vi "Calculate Node Width.vi"(11 "ClassInfo":T1[](array[typedef])) -> (3 "upper limit":i16)   [LabVIEW 2016, in "LV Object Event Registration Node.xnode"]
uses:
  LV Object Event Registration Node.xnode
  LOER_ClassInfo.ctl
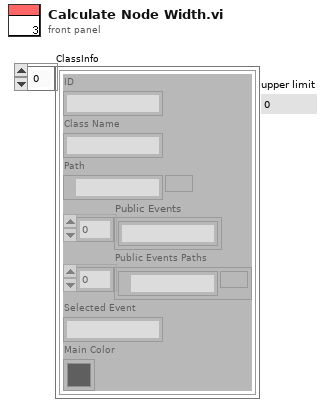
[diagram p1: front panel]
types:
  T1 = typedef "LV Object Event Registration Node.xnode/LOER_ClassInfo.ctl" = cluster{"ID":string, "Class Name":string, "Path":path, "Public Events":string[], "Public Events Paths":path[], "Selected Event":string, "Main Color":u32}
  T2 = cluster{"left":i16, "top":i16, "right":i16, "bottom":i16}
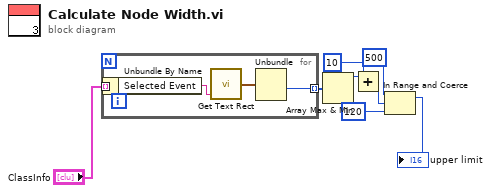
[diagram p0: block diagram]
diagram:
  n1 = for {
    tunnel: "ClassInfo" -> [w11] mode=indexing
    tunnel: [w9] -> w2 mode=indexing
    n2 = Unbundle By Name(w11) -> ("Selected Event"=w10:string)
    n3 = call <vilib>:"Get Text Rect.vi"("text"=w10) -> ("rect"=w12:T2)  [unwired: 8 in]
    n4 = Unbundle(w12) -> ("right"=w9:i16)  [unwired: 3 out]
  }
  n5 = Array Max & Min(array=w2) -> (max value=w4:i16)  [unwired: 3 out]
  n6 = Add(x=w4, y=i16 10) -> (x+y=w7:i16)
  n7 = In Range and Coerce(upper limit=i16 500, x=w7, lower limit=i16 120) -> (coerced(x)=→"upper limit":i16)  [unwired: 1 out]
